vi "Event Module Overrun.vi"(6 "Channel (Channel A)":enum16{"Channel A", "Channel B"}(ring), 7 "Event Module # (1)":u32=1 min=1 max=14, 8 "error in":errorcluster, 9 "Event Module Type (Digital I/O)":T1(ring), 10 "Node In":string, 11 "VISA resource name":refnum<visa-resource-name>) -> (0 "error out":errorcluster, 1 "Overrun?":bool, 2 "Node Out":string, 3 "VISA resource name out":refnum<visa-resource-name>, 4 "Command String":string)   [LabVIEW 2013, in "Keithley 2600 Series.lvlib"]
doc: "This VI is used to check if an event module has been overrun.\n\n<b>Functions and Attributes Used</b>\ndigio.trigger[n].overrun\ntsplink.trigger[n].overrun\nlan.trigger[n].overrun\ntrigger.blender[n].overrun\ntrigger.timer[n].overrun\nsmuX.trigger.arm.overrun\nsmuX.trigger.source.overrun\nsmuX.trigger.measure.overrun\nsmuX.trigger.endpulse.overrun"
uses:
  Keithley 2600 Series.lvlib
  Private/GlobalVariables.vi
panel:
  # "(c) 2008 Keithley Instruments, Inc.  ALL RIGHTS RESERVED."
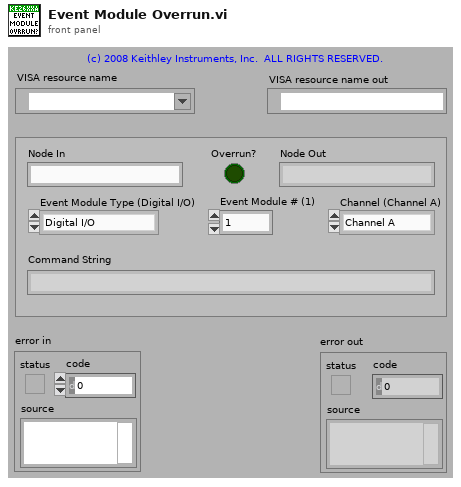
[diagram p1: front panel]
types:
  T1 = enum16{"Digital I/O", "TSP-Link", "LAN", "Blender", "Timer", "Arm", "Source", "Measure", "End Pulse"}
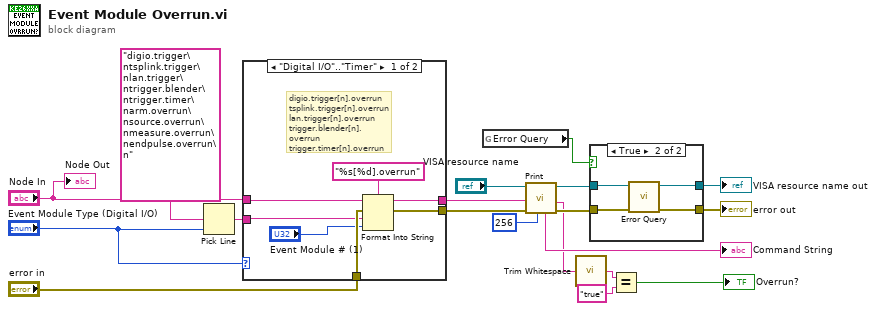
[diagram p0: block diagram]
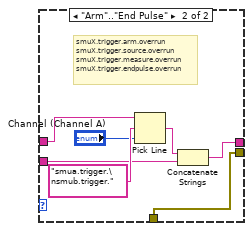
[diagram p3: hidden frame]
diagram:
  n1 = Pick Line(multi-line string="digio.trigger\ntsplink.trigger\nlan.trigger\ntrigger.blender\ntrigger.timer\narm.overrun\nsource.overrun\nmeasure.overrun\nendpulse.overrun\n", line index="Event Module Type (Digital I/O)") -> (output string=w15:string)  [unwired: 1 out]
  n2 = case shown="\"Digital I/O\"..\"Timer\"" "Event Module Type (Digital I/O)" {
    tunnel: "Node In" -> [w22 w31]
    tunnel: [w25 w28] -> w10
    tunnel: [w24 w27] -> w9
    tunnel: "error in" -> [w23 w27]
    tunnel: w15 -> [w21 w29]
    frame "Digital I/O".."Timer" {
      # "digio.trigger[n].overrun\ntsplink.trigger[n].overrun\nlan.trigger[n].overrun\ntrigger.blender[n].overrun\ntrigger.timer[n].overrun"
      n3 = Format Into String(format string="%s[%d].overrun", initial string=w22, error in=w23, w21, "Event Module # (1)") -> (resulting string=w25:string, error out=w24:errorcluster)
    }
    frame "Arm".."End Pulse" {
      # "smuX.trigger.arm.overrun\nsmuX.trigger.source.overrun\nsmuX.trigger.measure.overrun\nsmuX.trigger.endpulse.overrun"
      n4 = Pick Line(string ("")=w31, multi-line string="smua.trigger.\nsmub.trigger.", line index="Channel (Channel A)") -> (output string=w30:string)
      n5 = Concatenate Strings(w30, w29) -> (w28:string)
    }
  }
  n6 = global read "GlobalVariables.vi" "Error Query"() -> (w12:bool)
  n7 = call "Print.vi"("Byte Count (1024)"=u32 256, "error in (no error)"=w9, "Input"=w10, "VISA resource name"="VISA resource name") -> ("error out"=w5:errorcluster, "Output"=w4:string, "VISA resource name out"=w6:refnum<visa-resource-name>, "Command String"=→"Command String":string)  [unwired: 1 in, 3 out]
  n8 = call <vilib>:"Trim Whitespace.vi"("string"=w4) -> ("trimmed string"=w2:string)  [unwired: 1 in]
  n9 = case shown="True" w12 {
    tunnel: w6 -> [w35 w39]
    tunnel: w5 -> [w34 w38]
    tunnel: [w35 w37] -> w14
    tunnel: [w34 w36] -> w13
    frame False {
    }
    frame True {
      n10 = call "Error Query.vi"("error in (no error)"=w38, "VISA resource name"=w39) -> ("error out"=w36:errorcluster, "VISA resource name out"=w37:refnum<visa-resource-name>)  [unwired: 8 out]
    }
  }
  "VISA resource name out" <- w14
  "error out" <- w13
  n11 = Equal?(x=w2, y="true") -> (x = y?=→"Overrun?":bool)
  "Node Out" <- "Node In"
